vi "Reference Queue.vi"(5 "timeout in ms (-1)":i32=-1, 6 "Queue Name":string, 7 "Priority Message? (F)":bool, 8 "error in (no error)":errorcluster, 9 "Message Data":variant, 10 "Tasks":T1, 11 "VI Refnum":refnum<vi>) -> (0 "error out":errorcluster)   [LabVIEW 2019, in "Test.lvlib"]
doc: "Function to enqueue a Message in a Queue of other Module."
uses:
  Test.lvlib
  State Name.ctl
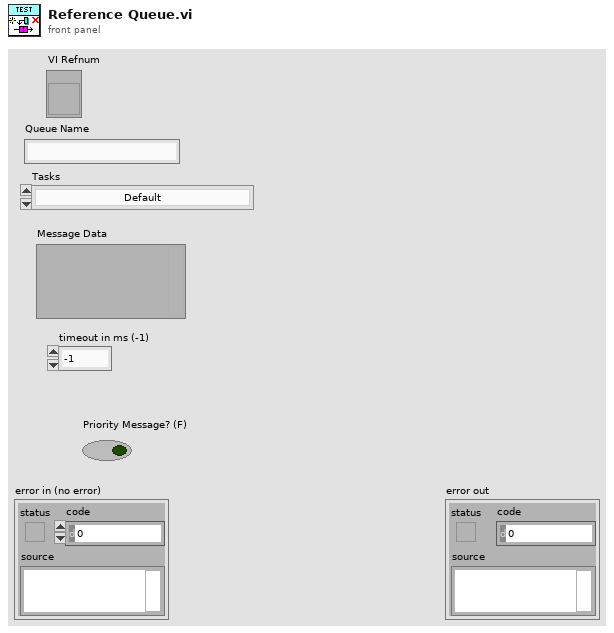
[diagram p1: front panel]
types:
  T1 = typedef "Test.lvlib/State Name.ctl" = enum16{"Default", "Initialize", "Re-Initialize", "Initialize Data", "Initialize Panel", "[Event Structure] Update Data", "Error", "Exit"}
  T2 = typedef "Message Queue Ref.ctl" = refnum<queue>
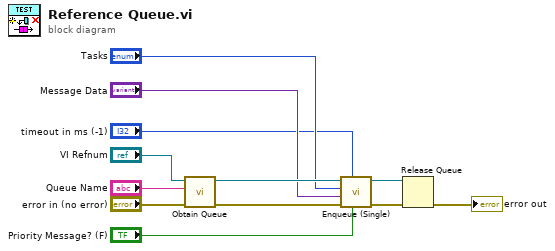
[diagram p0: block diagram]
diagram:
  n1 = call "Obtain Queue.vi"("error in (no error)"="error in (no error)", "Queue Name"="Queue Name", "VI Refnum"="VI Refnum") -> ("error out"=w8:errorcluster, "Message out"=w10:T2)  [unwired: 7 in]
  n2 = call "Enqueue (Single).vi"("Priority Message? Array"="Priority Message? (F)", "timeout in ms (-1)"="timeout in ms (-1)", "error in (no error)"=w8, "Message Data Array"="Message Data", "States"="Tasks", "Message Queue"=w10) -> ("error out"=w4:errorcluster, "Message Queue dub"=w5:T2)  [unwired: 4 in]
  n3 = Release Queue(queue=w5, error in (no error)=w4) -> (error out=→"error out":errorcluster)  [unwired: 1 in, 2 out]
